vi "StringToBuildVersion.vi"(10 "Version string":string="0.0.0.0") -> (2 "Version":T1)   [LabVIEW 2019]
uses:
  <vilib>/JKI/VIPM API/command-line/support/Version Info Cluster_vipm_api.ctl
  <vilib>/JKI/VIPM API/VIPM API_vipm_api.lvlib
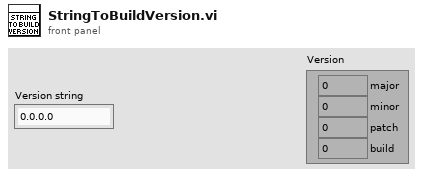
[diagram p1: front panel]
types:
  T1 = typedef "VIPM API_vipm_api.lvlib/Version Info Cluster_vipm_api.ctl" = cluster{"major":u32, "minor":u32, "patch":u32, "build":u32}
  T2 = cluster{"[0]":u32, "[1]":u32, "[2]":u32, "[3]":u32}
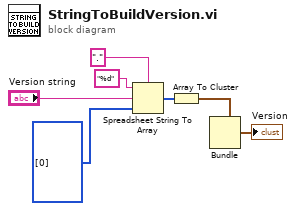
[diagram p0: block diagram]
diagram:
  n1 = Spreadsheet String To Array(delimiter (Tab)=".", format string="%d", spreadsheet string="Version string", array type (2D Dbl)=u32[] [0]) -> (array=w7:u32[])
  n2 = Array To Cluster(array=w7) -> (cluster=w4:T2)
  n3 = Bundle(cluster=w4) -> (→"Version":T2)  [unwired: 4 in]
